vi "Set Needle Valve.vi"(8 "error in (no error)":errorcluster, 10 "Needle Valve (%)":dbl min=0.0 max=100.0, 11 "Instrument.1820 in":refnum<class "Instrument.Oxford1820.lvclass">) -> (0 "error out":errorcluster, 2 "Response":string, 3 "Instrument.1820 in":refnum<class "Instrument.Oxford1820.lvclass">)   [LabVIEW 2019, in "Instrument.Oxford1820.lvclass"]
uses:
  Instrument.Oxford1820.lvclass
  C:/Program Files (x86)/National Instruments/LabVIEW 2019/user.lib/LevyLab/Levylab Instruments/SMOs/Instrument/Instrument.lvclass
  Typedefs/Instrument.Oxford1820.Commands-enum.ctl
  <userlib>/LevyLab/Instrument Framework/SMOs/Instrument/Instrument.lvclass/Instrument.ctl
  97883e26-1ce3-48ed-90c4-6daa8cf719e8.vi
  97883e26-1ce3-48ed-90c4-6daa8cf719e8.vi/a1d46c74-6d94-46ed-be88-04efa1ef93cb.vi
  97883e26-1ce3-48ed-90c4-6daa8cf719e8.vi/a1d46c74-6d94-46ed-be88-04efa1ef93cb.vi/90b59ab8-a335-4443-95d6-154de20b2a7b.vi
  <userlib>/LevyLab/Instrument Framework/SMOs/Instrument/API/Send and Receive.vi
  97883e26-1ce3-48ed-90c4-6daa8cf719e8.vi/a1d46c74-6d94-46ed-be88-04efa1ef93cb.vi/90b59ab8-a335-4443-95d6-154de20b2a7b.vi/ec1554c9-4b1a-47cd-aff6-1da852050cec.vi
  97883e26-1ce3-48ed-90c4-6daa8cf719e8.vi/a1d46c74-6d94-46ed-be88-04efa1ef93cb.vi/90b59ab8-a335-4443-95d6-154de20b2a7b.vi/5e080cdb-aae0-4c57-ab2c-75446a812738.vi
  <userlib>/LevyLab/Instrument Framework/SMOs/Instrument/API/Enum to String.vi
  <userlib>/LevyLab/Instrument Framework/SMOs/RemoteControl/API/Send and Receive.vi
  <vilib>/Utility/Data Type/Get Type Information.vi
  <vilib>/JDP Science/JSONtext/JSON text to Variant.vi
  <vilib>/JDP Science/JSONtext/LVClass Serializer/JSONtext LVClass Serializer.lvclass
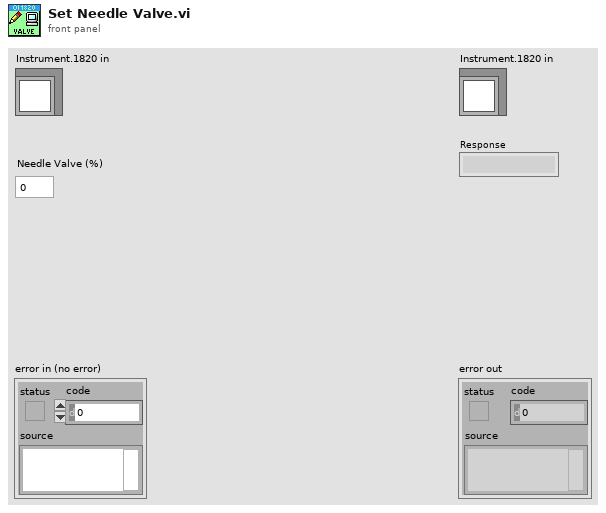
[diagram p1: front panel]
types:
  T1 = typedef "Instrument.Oxford1820.lvclass/Instrument.Oxford1820.Commands-enum.ctl" = enum16{"setAction", "setTarget", "setSwitchHeat", "setLambda", "setFillMode", "setNeedleValve", "setMagnetField", "getStatus", "getTarget", "getSwitchHeat", "getPSUField", "setSequenceStatus", "getMagnetField"}
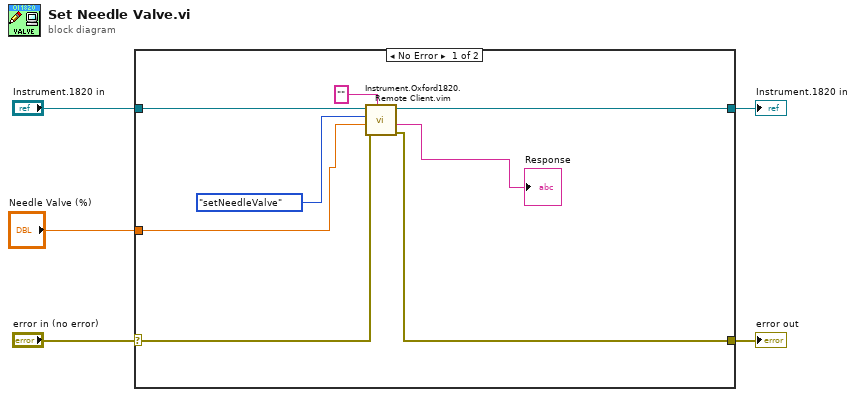
[diagram p0: block diagram]
diagram:
  n1 = case shown="No Error" "error in (no error)" {
    selector: "error in (no error)" -> [w12 w15]
    tunnel: [w7 w15] -> w4
    tunnel: [w6 w14] -> w2
    tunnel: "Instrument.1820 in" -> [w13 w14]
    tunnel: "Needle Valve (%)" -> [w10 _]
    frame No Error {
      n2 = call "Instrument.Oxford1820.Remote Client.vim"("Data Out type"="", "error in (no error)"=w12, "Data"=w10, "Commands"=Instrument.Oxford1820.Commands-enum."setNeedleValve", "Instrument.1820 in"=w13) -> ("error out"=w7:errorcluster, "Data out"=→"Response":string, "Instrument.1820 out"=w6:refnum<class "Instrument.Oxford1820.lvclass">)  [unwired: 4 in]
    }
    frame Error {
    }
  }
  "error out" <- w4
  "Instrument.1820 in" <- w2
